vi "Set Point.vi"(8 "error in (no error)":errorcluster, 9 "Output #":i32=1, 10 "Set point":dbl, 11 "Neocera Driver in":refnum<class "Neocera Driver.lvclass">) -> (0 "error out":errorcluster, 3 "Neocera Driver out":refnum<class "Neocera Driver.lvclass">)   [LabVIEW 2021, in "Neocera Driver.lvclass"]
uses:
  Neocera Driver.lvclass
  C:/GitHub/NHMFL_Core/Libraries/Instruments/VISA Instrument/VISA Instrument.lvclass
  VISA Instrument/VISA Instrument.lvclass/VISA Instrument.ctl
  VISA Instrument/Read VISA resource.vi
  VISA Instrument/Write VISA resource.vi
  Neocera Driver.lvclass/Neocera Driver.ctl
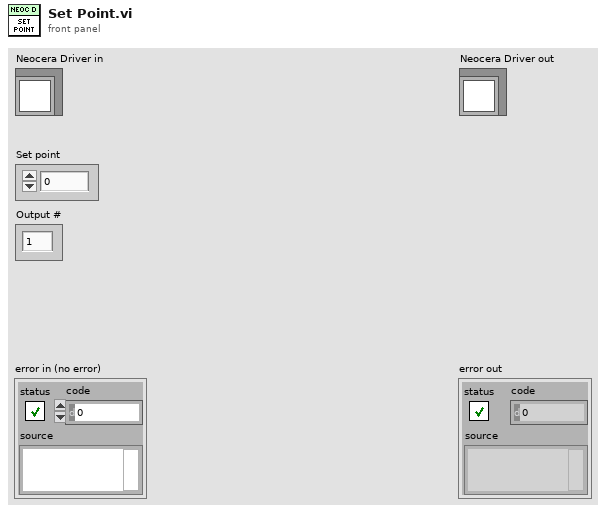
[diagram p1: front panel]
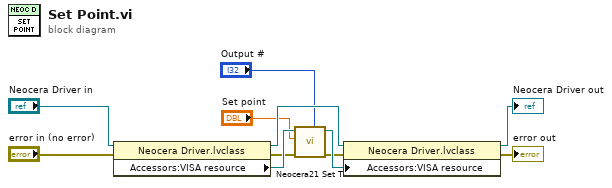
[diagram p0: block diagram]
diagram:
  n1 = property class="Neocera Driver.lvclass"(reference="Neocera Driver in", error in="error in (no error)") -> (reference out=w11:refnum<class "Neocera Driver.lvclass">, error out=w3:errorcluster, "Accessors:VISA resource"=w6:refnum<visa-resource-name>)
  n2 = call "Neocera21 Set T.vi"("Channel"="Output #", "error in (no error)"=w3, "Set T"="Set point", "VISA Resource Name"=w6) -> ("error out"=w4:errorcluster, "VISA Resource Name Out"=w5:refnum<visa-resource-name>)  [unwired: 6 in]
  n3 = property class="Neocera Driver.lvclass"(reference=w11, error in=w4, "Accessors:VISA resource"=w5) -> (reference out=→"Neocera Driver out":refnum<class "Neocera Driver.lvclass">, error out=→"error out":errorcluster)
